vi "midioutshortmsg.vi"(2 "Data":i32 format="%.0x", 3 "MIDI output handle":i32) -> (0 "Win32 error code":i32, 1 "Duplicate MIDI output handle":i32)   [LabVIEW 2016]
uses:
  winmm.dll
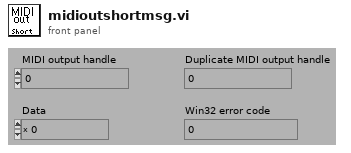
[diagram p1: front panel]
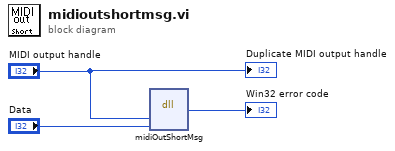
[diagram p0: block diagram]
diagram:
  n1 = dll-call lib="winmm.dll" fn="midiOutShortMsg"("hmidiout"="MIDI output handle", "data"="Data") -> (→"Win32 error code":i32)  [unwired: 5 in, 2 out]
  "Duplicate MIDI output handle" <- "MIDI output handle"
